vi "合并矩形（TB）.vi"(10 "矩形B":T1, 11 "矩形A":T1) -> (3 "合并矩形":T1)   [LabVIEW 2011]
uses:
  RectTB.ctl
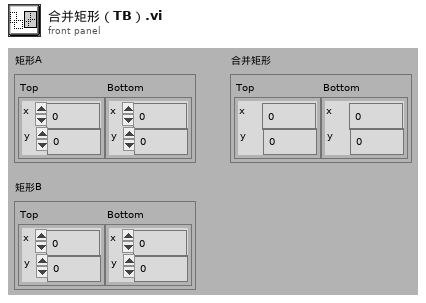
[diagram p1: front panel]
types:
  T1 = typedef "RectTB.ctl" = cluster{"Top":cluster{"x":i16, "y":i16}, "Bottom":cluster{"x":i16, "y":i16}}
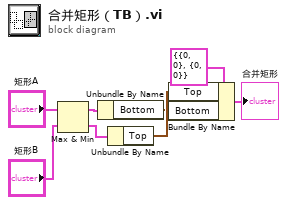
[diagram p0: block diagram]
diagram:
  n1 = Max & Min(x="矩形A", y="矩形B") -> (max(x,y)=w5:T1, min(x,y)=w6:T1)
  n2 = Unbundle By Name(w5) -> ("Bottom"=w3:cluster{"x":i16, "y":i16})
  n3 = Unbundle By Name(w6) -> ("Top"=w4:cluster{"x":i16, "y":i16})
  n4 = Bundle By Name(cluster=T1 {"Top"={"x"=0, "y"=0}, "Bottom"={"x"=0, "y"=0}} ("合并矩形"), "Top"=w4, "Bottom"=w3) -> (→"合并矩形":T1)
